vi "SensorReadOneCircle.vi"(0 "controller":refnum<k24>, 1 "VISA resource name":refnum<visa-resource-name>="COM4", 2 "StartPoint":T1 {"X" format="%#.5g"; "Y" format="%#.5g"; "Z" format="%#.5g"}, 3 "error out":errorcluster) -> (7 "controller out":refnum<k24>, 8 "VISA resource name out":refnum<visa-resource-name>, 9 "AverageReading":dbl, 10 "error out 2":errorcluster)   [LabVIEW 2016]
uses:
  Control/Coordinate.ctl
  C:/Users/TTUHEP/Documents/LabVIEW/Other Models/2010/Bin/Aerotech.A3200.dll
  Other Models/2010/Bin/Aerotech.A3200.dll
  Other Models/2010/Status/ControllerDiagPacket.ctl
  Other Models/2010/Status/AxisDiagPacket.ctl
  <vilib>/Instr/_visa.llb/VISA Configure Serial Port (Instr).vi
panel:
  out "Boolean":bool=TRUE
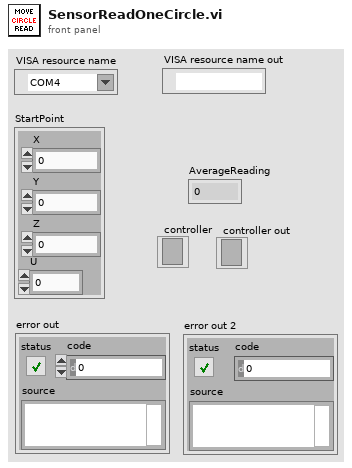
[diagram p1: front panel]
types:
  T1 = typedef "Coordinate.ctl" = cluster{"X":dbl, "Y":dbl, "Z":dbl, "U":dbl}
  T2 = typedef "ControllerDiagPacket.ctl" = cluster{"Number of Diag Packets":i32, "Axes":T3[], "error":errorcluster}
  T3 = typedef "AxisDiagPacket.ctl" = cluster{"Axis Name":string, "Analog Input 0":dbl, "Analog Input 1":dbl, "Axis Fault (num)":i32, "Axis Fault (str)":string, "Axis Fault (bits)":cluster{"AmplifierFault":bool, "AmplifierTemperatureFault":bool, "CcwEndOfTravelLimitFault":bool, "CcwSoftwareLimitFault":bool, "CommunicationLostFault":bool, "CwEndOfTravelLimitFault":bool, "CwSoftwareLimitFault":bool, "EmergencyStopFault":bool, "EncoderFault":bool, "ExternalFault":bool, "FeedbackScalingFault":bool, "GantryMisalignFault ":bool, "HallSensorFault":bool, "InPositionTimeoutFault":bool, "InternalFault":bool, "MarkerSearchFault":bool, "MaxVelocityCommandFault":bool, "MissedInterruptFault":bool, "MotorTemperatureFault":bool, "None":bool, "OverCurrentFault":bool, "PositionErrorFault":bool, "PositionFeedbackFault":bool, "PowerSupplyFault":bool, "ProbeInputFault":bool, "SafeZoneFault":bool, "VelocityErrorFault":bool, "VelocityFeedbackFault":bool, "VoltageClampFault":bool}, "Axis Status (num)":i32, "Axis Status (str)":string, "Axis Status (bits)":cluster{"BacklashActive":bool, "CalibrationEnabled1D":bool, "CalibrationEnabled2D":bool, "CommandValid":bool, "DriveAbortPending":bool, "DrivePending":bool, "Enabling":bool, "GainMappingEnabled":bool, "GantryAligned":bool, "GantryRealigning":bool, "Homed":bool, "Homing":bool, "IFOVEnabled":bool, "JogGenerating":bool, "Jogging":bool, "JoystickControl":bool, "MasterSlaveControl":bool, "MotionBlocked":bool, "MotionClamped":bool, "MoveDone":bool, "None":bool, "NotVirtual":bool, "Profiling":bool, "Stability0":bool, "Stability1":bool, "TrajectoryFiltering":bool, "WaitDone":bool}, "Current Command":sgl, "Current Error":sgl, "Current Feedback":sgl, "Digital Inputs":i32, "Digital Outputs":i32, "Drive Status":i32, "Drive Status (str)":string, "Drive Status (bits)":cluster{"AccelerationPhase":bool, "AutofocusActive":bool, "BrakeOutput":bool, "CcwEndOfTravelLimitInput":bool, "CosineEncoderError":bool, "CurrentClamp":bool, "CwEndOfTravelLimitInput":bool, "DecelerationPhase":bool, "DualLoopActive":bool, "EmergencyStopInput":bool, "Enabled":bool, "EncoderClipping":bool, "GalvoCalibrationEnabled":bool, "GalvoPowerCorrection":bool, "HallAInput":bool, "HallBInput":bool, "HallCInput":bool, "HighResolutionMode":bool, "HomeLimitInput":bool, "InPosition":bool, "InPosition2":bool, "MarkerInput":bool, "MarkerLatch":bool, "MoveActive":bool, "NoMotorSupply":bool, "None":bool, "PowerLimiting":bool, "ProgrammingFlash":bool, "ProgrammingMXH":bool, "PSOHaltLatch":bool, "ServoControl":bool, "SineEncoderError":bool}, "Position Feedback Auxiliary":dbl, "Position Command":dbl, "Position Error":dbl, "Position Feedback":dbl, "Program Position Command":dbl, "Program Position Error":dbl, "Program Position Feedback":dbl, "Velocity Command":dbl, "Velocity Error":dbl, "Velocity Feedback":dbl}
  T4 = cluster{"ControllerDiagPacket":T2, "read buffer":string}
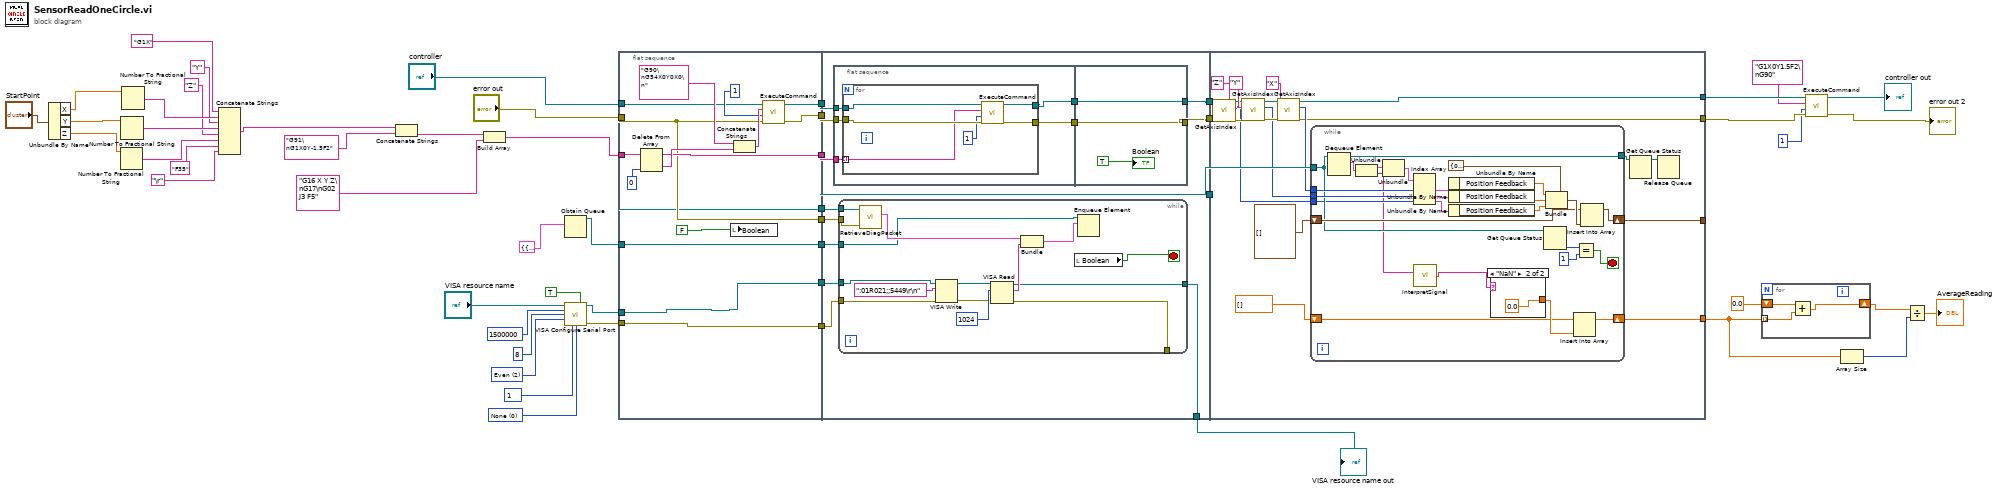
[diagram p0: block diagram]
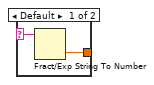
[diagram p2: hidden frame]
diagram:
  w26 = u16 0 items=["None"=0, "XON/XOFF"=1, "RTS/CTS"=2, "DTR/DSR"=4] ("flow control")
  w27 = u16 10 items=["1"=10, "1.5"=15, "2.0"=20] ("stop bits")
  w28 = u16 2 items=["None", "Odd", "Even", "Mark", "Space"] ("parity")
  n1 = Unbundle By Name("StartPoint") -> ("X"=w41:dbl, "Y"=w6:dbl, "Z"=w31:dbl)
  n2 = Number To Fractional String(number=w31) -> (F-format string=w32:string)  [unwired: 3 in]
  n3 = Number To Fractional String(number=w6) -> (F-format string=w39:string)  [unwired: 3 in]
  n4 = Number To Fractional String(number=w41) -> (F-format string=w40:string)  [unwired: 3 in]
  n5 = Concatenate Strings("G1X", w40, "Y", w39, "Z", w32, "F35", "\r") -> (w5:string)
  n6 = Concatenate Strings(w5, "G91\nG1X0Y-1.5F2") -> (w3:string)
  n7 = Build Array(w3, "G16 X Y Z\nG17\nG02 J3 F5") -> (w36:string[])
  n8 = Obtain Queue(element data type=cluster{"ControllerDiagPacket":T2, string} {"ControllerDiagPacket"={"Number of Diag Packets"=0, "Axes"=[], "error"={"status"=FALSE, "code"=0, "source"=""}}, ""}) -> (queue out=w34:refnum<queue>)  [unwired: 4 in, 2 out]
  n9 = call-poly "VISA Configure Serial Port"("VISA resource name"="VISA resource name", "Enable Termination\nChar (T)"=TRUE, "baud rate (9600)"=u32 1500000 ("baud rate"), "data bits (8)"=u16 8 ("data bits"), "parity (0:none)"=w28, "stop bits (10: 1 bit)"=w27, "flow control (0:none)"=w26) -> ("VISA resource name out"=w23:refnum<visa-resource-name>, "error out"=w22:errorcluster)  [unwired: 7 in]
  n10 = flat-sequence {
    tunnel: [w62] -> w53
    tunnel: [w66] -> w52
    tunnel: [w67] -> w51
    tunnel: w36 -> [w68]
    tunnel: [w56] -> w50
    tunnel: [w57] -> w49
    tunnel: w34 -> [w60]
    tunnel: [w60] -> w48
    tunnel: [w55] -> w47
    tunnel: [w54] -> w46
    tunnel: "error out" -> [w57]
    tunnel: "controller" -> [w56]
    tunnel: w23 -> [w55]
    tunnel: w22 -> [w54]
    tunnel: [w76] -> w45
    tunnel: w53 -> [w70]
    tunnel: w52 -> [w72]
    tunnel: w51 -> [w71]
    tunnel: w50 -> [w80]
    tunnel: w49 -> [w81]
    tunnel: w48 -> [w79]
    tunnel: [w79] -> w44
    tunnel: w47 -> [w78]
    tunnel: w46 -> [w77]
    tunnel: [w73] -> w43
    tunnel: [w69] -> w20
    tunnel: w45 -> [w118]
    tunnel: w44 -> [w131]
    tunnel: [w120] -> w17
    tunnel: [w119] -> _
    tunnel: w43 -> [w117]
    tunnel: [w112] -> w13
    tunnel: [w111] -> w12
    frame #0 {
      n11 = Delete From Array(array=w68, index=0) -> (deleted portion=w63:string, array with subset deleted=w62:string[])  [unwired: 1 in]
      n12 = local write "Boolean"(FALSE) -> ()
      n13 = Concatenate Strings("G90\nG54X0Y0X0\n", w63) -> (w61:string)
      n14 = call "ExecuteCommand.vi"("error in (no error)"=w57, "taskId"=1, "Command Code"=w61, "controller in"=w56) -> ("error out"=w67:errorcluster, "controller out"=w66:refnum<k24>)  [unwired: 5 in, 1 out]
    }
    frame #1 {
      n15 = flat-sequence {
        tunnel: [w86] -> w75
        tunnel: [w85] -> w74
        tunnel: w72 -> [w84]
        tunnel: w71 -> [w83]
        tunnel: w70 -> [w82]
        tunnel: [w94] -> w76
        tunnel: w75 -> [w94]
        tunnel: w74 -> [w93]
        tunnel: [w93] -> w73
        frame #0 {
          n16 = for {
            tunnel: w82 -> [w90] mode=indexing
            tunnel: w84 -> [w91]
            tunnel: w83 -> [w92]
            tunnel: [w88] -> w86
            tunnel: [w87] -> w85
            n17 = call "ExecuteCommand.vi"("error in (no error)"=w92, "taskId"=1, "Command Code"=w90, "controller in"=w91) -> ("error out"=w88:errorcluster, "controller out"=w87:refnum<k24>)  [unwired: 5 in, 1 out]
          }
        }
        frame #1 {
          "Boolean" <- TRUE
        }
      }
      n18 = while {
        tunnel: w80 -> [w110]
        tunnel: w81 -> [w109]
        tunnel: w79 -> [w103]
        tunnel: w78 -> [w99]
        tunnel: w77 -> [w98]
        tunnel: [w102] -> w69
        tunnel: [w101] -> _
        stop <- w104 stop-if-true
        n19 = call "RetrieveDiagPacket.vi"("error in (no error)"=w109, "Controller In"=w110) -> ("ControllerDiagPacket"=w107:T2)  [unwired: 7 in, 2 out]
        n20 = VISA Write(VISA resource name=w99, write buffer=":01R021;;5449\r\n" ("Command"), error in (no error)=w98) -> (VISA resource name out=w96:refnum<visa-resource-name>, error out=w97:errorcluster)  [unwired: 1 out]
        n21 = VISA Read(VISA resource name=w96, byte count=u32 1024, error in (no error)=w97) -> (VISA resource name out=w102:refnum<visa-resource-name>, read buffer=w106:string, error out=w101:errorcluster)  [unwired: 1 out]
        n22 = Bundle("ControllerDiagPacket"=w107, "read buffer"=w106) -> (w105:T4)  [unwired: 1 in]
        n23 = local read "Boolean"() -> (w104:bool)
        n24 = Enqueue Element(queue=w103, element=w105) -> ()  [unwired: 2 in, 3 out]
      }
    }
    frame #2 {
      n25 = call "GetAxisIndex.vi"("error in (no error)"=w118, "axis name"="Z", "controller in"=w117) -> ("error out"=w115:errorcluster, "axis index"=w113:i32, "controller out"=w116:refnum<k24>)  [unwired: 6 in]
      n26 = call "GetAxisIndex.vi"("error in (no error)"=w115, "axis name"="Y", "controller in"=w116) -> ("error out"=w129:errorcluster, "axis index"=w125:i32, "controller out"=w130:refnum<k24>)  [unwired: 6 in]
      n27 = call "GetAxisIndex.vi"("error in (no error)"=w129, "axis name"="X", "controller in"=w130) -> ("error out"=w111:errorcluster, "axis index"=w126:i32, "controller out"=w112:refnum<k24>)  [unwired: 6 in]
      n28 = while {
        tunnel: w126 -> [w156]
        tunnel: w125 -> [w155]
        shift-right: [w148] -> w119
        shift-left: cluster{"X":dbl, "Y":dbl, "Y 2":dbl}[] [] -> [w146]
        tunnel: [w147] -> w123
        tunnel: w131 -> [w142]
        shift-right: [w137] -> w120
        shift-left: dbl[] [] -> [w138]
        tunnel: w113 -> [w136]
        stop <- w144 stop-if-true
        n29 = Dequeue Element(queue=w142) -> (queue out=w147:refnum<queue>, element=w141:cluster{"ControllerDiagPacket":T2, string})  [unwired: 2 in, 2 out]
        n30 = Unbundle(w141) -> ("ControllerDiagPacket"=w140:T2, w133:string)
        n31 = Unbundle(w140) -> ("Axes"=w157:T3[])  [unwired: 2 out]
        n32 = Index Array(array=w157, index #1=w156, index #2=w155, index #3=w136) -> (element #1=w154:T3, element #2=w153:T3, element #3=w135:T3)
        n33 = call "InterpretSignal.vi"("String in"=w133) -> ("String out"=w132:string)
        n34 = Unbundle By Name(w154) -> ("Position Feedback"=w151:dbl)
        n35 = Unbundle By Name(w153) -> ("Position Feedback"=w150:dbl)
        n36 = Unbundle By Name(w135) -> ("Position Feedback"=w134:dbl)
        n37 = case shown="\"NaN\"" w132 {
          selector: w132 -> [w159 _]
          tunnel: [w158 0.0] -> w139
          frame Default {
            n38 = Fract/Exp String To Number(string=w159) -> (number=w158:dbl)  [unwired: 3 in, 1 out]
          }
          frame "NaN" {
          }
        }
        n39 = Get Queue Status(queue=w142) -> (# elements in queue=w145:i32)  [unwired: 2 in, 7 out]
        n40 = Bundle(cluster=cluster{"X":dbl, "Y":dbl, "Z":dbl} {"X"=0.0, "Y"=0.0, "Z"=0.0}, "X"=w151, "Y"=w150, "Z"=w134) -> (w149:cluster{"X":dbl, "Y":dbl, "Z":dbl})
        n41 = Insert Into Array(array=w138, new element=w139) -> (w137:dbl[])  [unwired: 1 in]
        n42 = Equal?(x=w145, y=1) -> (x = y?=w144:bool)
        n43 = Insert Into Array(array=w146, new element=w149) -> (w148:cluster{"X":dbl, "Y":dbl, "Y 2":dbl}[])  [unwired: 1 in]
      }
      n44 = Get Queue Status(queue=w123) -> (queue out=w122:refnum<queue>)  [unwired: 2 in, 7 out]
      n45 = Release Queue(queue=w122) -> ()  [unwired: 2 in, 3 out]
    }
  }
  n46 = for {
    tunnel: w17 -> [w162] mode=indexing
    shift-right: [w161] -> w16
    shift-left: 0.0 -> [w163]
    n47 = Add(x=w163, y=w162) -> (x+y=w161:dbl)
  }
  n48 = call "ExecuteCommand.vi"("error in (no error)"=w12, "taskId"=1, "Command Code"="G1X0Y1.5F2\nG90", "controller in"=w13) -> ("error out"=→"error out 2":errorcluster, "controller out"=→"controller out":refnum<k24>)  [unwired: 5 in, 1 out]
  n49 = Array Size(array=w17) -> (size(s)=w15:i32)
  n50 = Divide(x=w16, y=w15) -> (x/y=→"AverageReading":dbl)
  "VISA resource name out" <- w20
